vi "getPluginListFromUsi.vi"(4 "error in (no error)":errorcluster) -> (0 "error out":errorcluster, 3 "plugins":T1[](array[typedef]))   [LabVIEW 2017]
uses:
  <vilib>/Platform/storage/Storage.llb/usiPluginDescription.ctl
  <vilib>/Platform/storage/Storage.llb/__loadPropString.vi
  <vilib>/Platform/storage/Storage.llb/__loadPropRefList.vi
  <vilib>/Platform/storage/Storage.llb/__loadPropInt32.vi
  <resource>/objmgr/Storage.rc
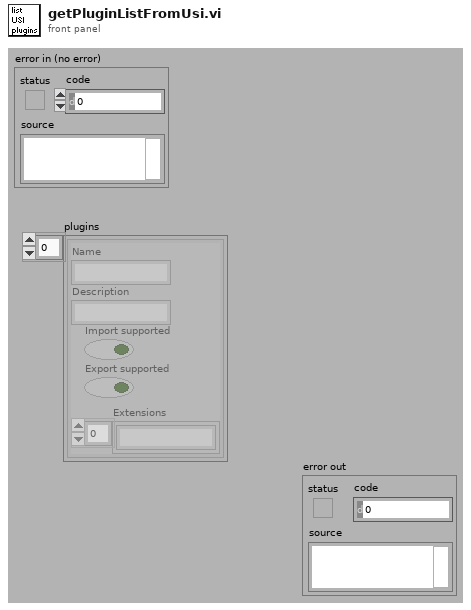
[diagram p1: front panel]
types:
  T1 = typedef "usiPluginDescription.ctl" = cluster{"Name":string, "Description":string, "Import supported":bool, "Export supported":bool, "Extensions":string[]}
  T2 = cluster{"Value":string, "Value":string, bool, bool, string[]}
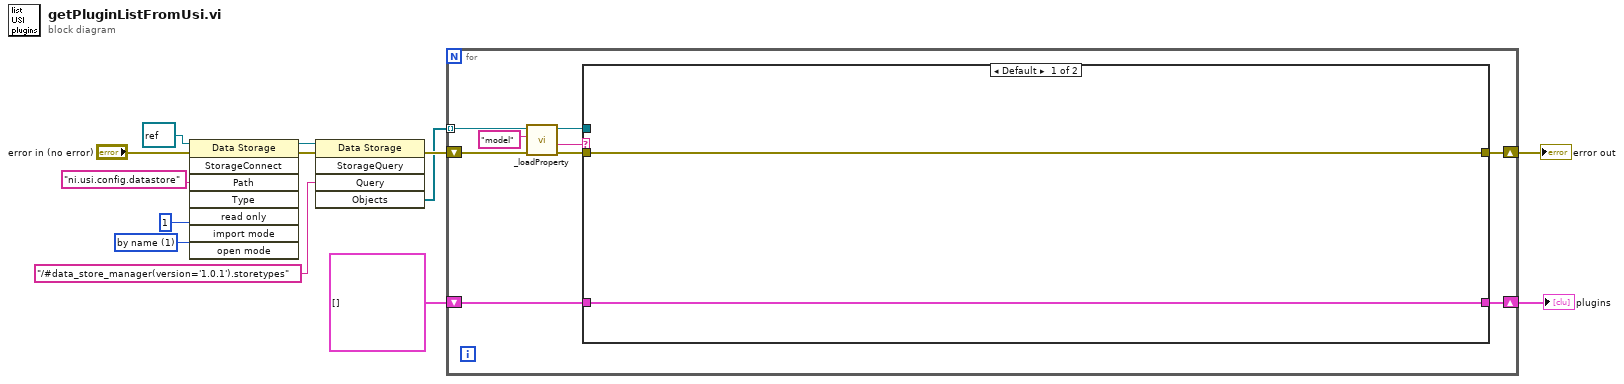
[diagram p0: block diagram]
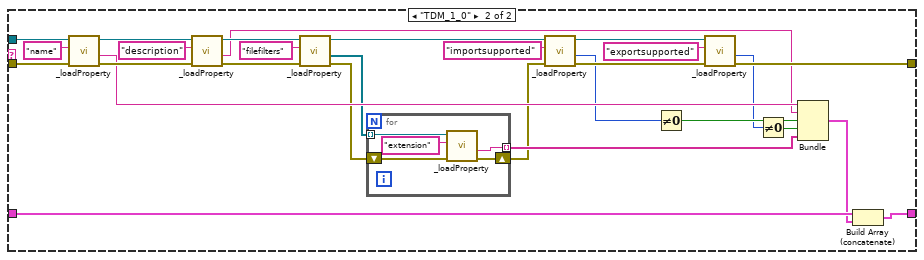
[diagram p2: hidden frame]
diagram:
  w1 = 1 items=["by param", "by name"] ("open mode")
  n1 = invoke class="Data Storage" method="StorageConnect"(reference=refnum<k20> refnum, error in="error in (no error)", "Path"="ni.usi.config.datastore", "import mode"=1, "open mode"=w1) -> (reference out=w12:refnum<k20>, error out=w8:errorcluster)  [unwired: 3 in, 6 out]
  n2 = invoke class="Data Storage" method="StorageQuery"(reference=w12, error in=w8, "Query"="/#data_store_manager(version='1.0.1').storetypes") -> (error out=w7:errorcluster, "Objects"=w6:refnum<k20>[])  [unwired: 2 in, 3 out]
  n3 = for {
    tunnel: w6 -> [w20] mode=indexing
    shift-right: [w22] -> w5
    shift-left: w7 -> [w19]
    shift-right: [w14] -> w2
    shift-left: T1[] [] -> [w15]
    n4 = call-poly <vilib>:"_loadProperty.vi"("error in (no error)"=w19, "Property name"="model", "storage refnum"=w20) -> ("error out"=w18:errorcluster, "Value"=w16:string, "dup storage refnum"=w17:refnum<k20>)  [unwired: 6 out]
    n5 = case shown="Default" w16 {
      tunnel: [w24 w41] -> w22
      tunnel: w18 -> [w24 w29]
      tunnel: w17 -> [_ w28]
      tunnel: w15 -> [w23 w27]
      tunnel: [w23 w25] -> w14
      frame Default {
      }
      frame "TDM_1_0" {
        n6 = call-poly <vilib>:"_loadProperty.vi"("error in (no error)"=w29, "Property name"="name", "storage refnum"=w28) -> ("error out"=w50:errorcluster, "Value"=w40:string, "dup storage refnum"=w49:refnum<k20>)  [unwired: 6 out]
        n7 = call-poly <vilib>:"_loadProperty.vi"("error in (no error)"=w50, "Property name"="description", "storage refnum"=w49) -> ("error out"=w46:errorcluster, "Value"=w39:string, "dup storage refnum"=w47:refnum<k20>)  [unwired: 6 out]
        n8 = call-poly <vilib>:"_loadProperty.vi"("error in (no error)"=w46, "Property name"="filefilters", "storage refnum"=w47) -> ("error out"=w35:errorcluster, "Value"=w36:refnum<k20>[], "dup storage refnum"=w37:refnum<k20>)  [unwired: 6 out]
        n9 = for {
          tunnel: w36 -> [w57] mode=indexing
          tunnel: [w55] -> w38 mode=indexing
          shift-right: [w53] -> w34
          shift-left: w35 -> [w54]
          n10 = call-poly <vilib>:"_loadProperty.vi"("error in (no error)"=w54, "Property name"="extension", "storage refnum"=w57) -> ("error out"=w53:errorcluster, "Value"=w55:string)  [unwired: 7 out]
        }
        n11 = call-poly <vilib>:"_loadProperty.vi"("error in (no error)"=w34, "Property name"="importsupported", "storage refnum"=w37) -> ("error out"=w43:errorcluster, "Value"=w33:i32, "dup storage refnum"=w42:refnum<k20>)  [unwired: 6 out]
        n12 = Not Equal To 0?(x=w33) -> (x != 0?=w32:bool)
        n13 = call-poly <vilib>:"_loadProperty.vi"("error in (no error)"=w43, "Property name"="exportsupported", "storage refnum"=w42) -> ("error out"=w41:errorcluster, "Value"=w30:i32)  [unwired: 7 out]
        n14 = Not Equal To 0?(x=w30) -> (x != 0?=w31:bool)
        n15 = Bundle("Value"=w40, "Value"=w39, w32, w31, w38) -> (w26:T2)  [unwired: 1 out]
        n16 = Build Array (concatenate)(w27, w26) -> (w25:T1[])
      }
    }
  }
  "error out" <- w5
  "plugins" <- w2
